vi "Stop Measurements Command.vi"(8 "error in (no error)":errorcluster, 10 "Measurement Controller":string, 11 "Monitor-Pulse in":refnum<class "Application Controller.lvclass">) -> (0 "error out":errorcluster, 3 "Monitor-Pulse out":refnum<class "Application Controller.lvclass">)   [LabVIEW 2018, in "Application Controller.lvclass"]
uses:
  Controllers/Application Controller/Application Controller.lvclass
  Controllers/Process Controller/Request type.ctl
  Controllers/Process Controller Messages/Stop Measurements Msg/Stop Measurements Msg.lvclass/Stop Measurements Msg.ctl
  <vilib>/ActorFramework/Message Enqueuer/Message Enqueuer.lvclass/Message Enqueuer.ctl
  <vilib>/ActorFramework/Message Enqueuer/Enqueue.vi
  Controllers/Process Controller Messages/Stop Measurements Msg/Stop Measurements Msg.lvclass
  C:/Program Files/National Instruments/LabVIEW 2018/vi.lib/ActorFramework/Message/Message.lvclass
  <vilib>/ActorFramework/Message Priority Queue/Priority Enqueue.vi
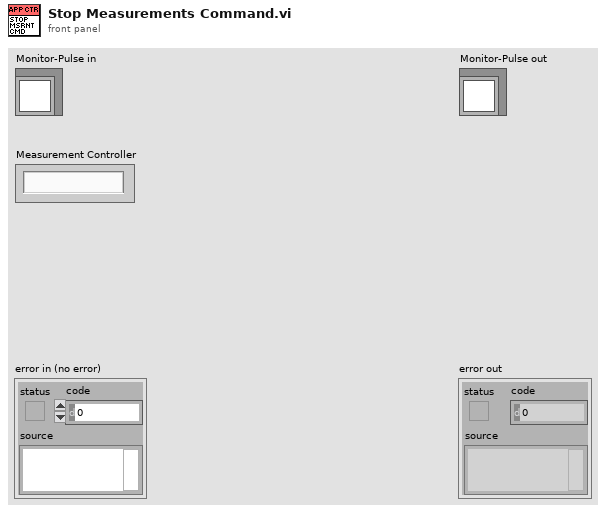
[diagram p1: front panel]
types:
  T1 = typedef "Request type.ctl" = enum16{"Process complete", "User command", "Auto-restart", "Error"}
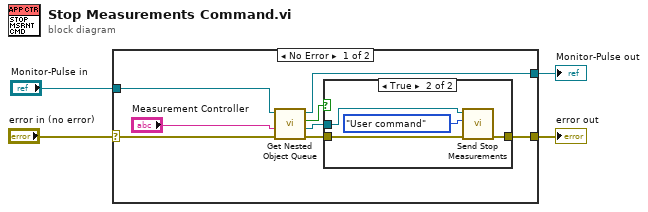
[diagram p0: block diagram]
diagram:
  n1 = case shown="No Error" "error in (no error)" {
    selector: "error in (no error)" -> [w7 w19]
    tunnel: [w5 w19] -> w3
    tunnel: [w9 w18] -> w1
    tunnel: "Monitor-Pulse in" -> [w10 w18]
    frame No Error {
      n2 = call-dynamic "Get Nested Object Queue.vi"("error in (no error)"=w7, "Name"="Measurement Controller", "Measure Object in"=w10) -> ("error out"=w6:errorcluster, "Object Enqueuer"=w11:refnum<class "Message Enqueuer.lvclass">, "Found?"=w8:bool, "Measure Object out"=w9:refnum<class "Application Controller.lvclass">)  [unwired: 5 in]
      n3 = case shown="True" w8 {
        tunnel: w11 -> [_ w17]
        tunnel: w6 -> [w13 w16]
        tunnel: [w13 w15] -> w5
        frame False {
        }
        frame True {
          n4 = call "Send Stop Measurements.vi"("error in (no error)"=w16, "Request type"=Request_type."User command", "Message Enqueuer"=w17) -> ("error out"=w15:errorcluster)  [unwired: 7 in, 1 out]
        }
      }
    }
    frame Error {
    }
  }
  "error out" <- w3
  "Monitor-Pulse out" <- w1
